vi "chart series set marker type.vi"(8 "error in (no error)":errorcluster, 10 "type":T1 items=["LXW_CHART_MARKER_AUTOMATIC", "LXW_CHART_MARKER_NONE", "LXW_CHART_MARKER_SQUARE", "LXW_CHART_MARKER_DIAMOND", "LXW_CHART_MARKER_TRIANGLE", "LXW_CHART_MARKER_X", "LXW_CHART_MARKER_STAR", "LXW_CHART_MARKER_SHORT_DASH", "LXW_CHART_MARKER_LONG_DASH", "LXW_CHART_MARKER_CIRCLE", "LXW_CHART_MARKER_PLUS"], 11 "series":u32) -> (0 "error out":errorcluster)   [LabVIEW 2015, in "xlsxwriter.lvlib"]
doc: "void chart_series_set_marker_type(lxw_chart_series series, uint8_t type);"
uses:
  xlsxwriter.lvlib
  Controls/lxw_chart_marker_type.ctl
  xlsxwriter.dll
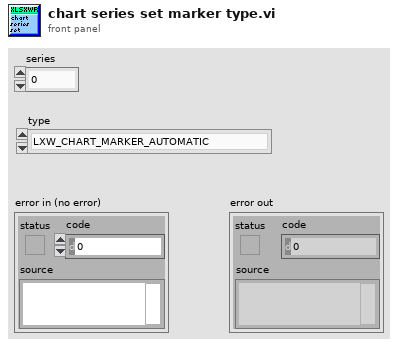
[diagram p1: front panel]
types:
  T1 = typedef "lxw_chart_marker_type.ctl" = u8
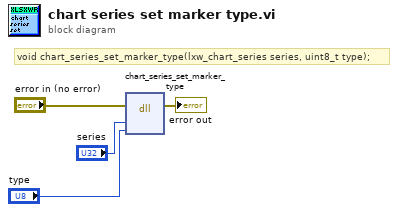
[diagram p0: block diagram]
diagram:
  # "void chart_series_set_marker_type(lxw_chart_series series, uint8_t type);"
  n1 = dll-call lib="C:/Users/WDAGUtilityAccount/Desktop/Labview_Example-win32/xlsxwriter.*" fn="chart_series_set_marker_type"(error in="error in (no error)", "series"="series", "type"="type") -> (error out=→"error out":errorcluster)  [unwired: 5 in, 1 out]
